vi "setParents.vi"(8 "error in (no error)":errorcluster, 10 "Parents":refnum<data-value>[](array[refnum]), 11 "MultiTreeNode in":refnum<class "MultiTreeNode.lvclass">) -> (0 "error out":errorcluster, 3 "MultiTreeNode out":refnum<class "MultiTreeNode.lvclass">)   [LabVIEW 2014, in "MultiTree.lvlib" / "MultiTreeNode.lvclass"]
uses:
  <userlib>/AdvancedDataStructures/ClassBased/MultiTreeNode/MultiTreeNode.lvclass
  <userlib>/AdvancedDataStructures/ClassBased/MultiTreeNode/MultiTreeNode.lvclass/MultiTreeNode.ctl
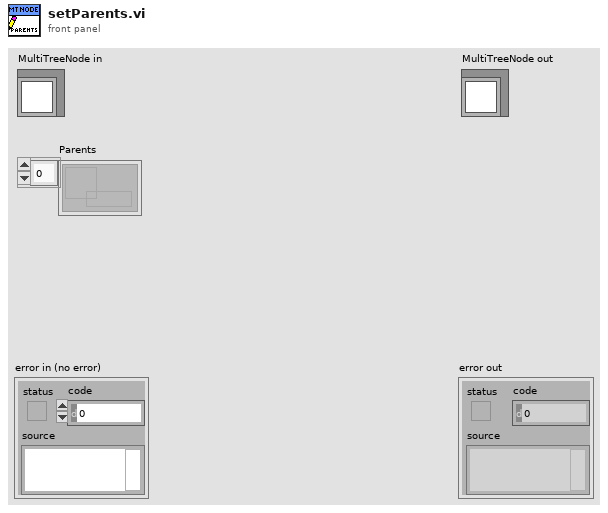
[diagram p1: front panel]
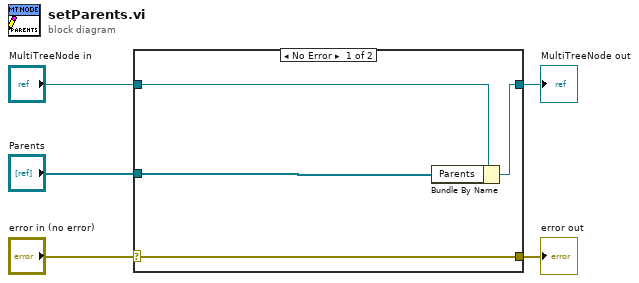
[diagram p0: block diagram]
diagram:
  n1 = case shown="No Error" "error in (no error)" {
    selector: "error in (no error)" -> [w9 w10]
    tunnel: [w9 w10] -> w4
    tunnel: [w7 w11] -> w2
    tunnel: "MultiTreeNode in" -> [w8 w11]
    tunnel: "Parents" -> [w6 _]
    frame No Error {
      n2 = Bundle By Name(cluster=w8, "Parents"=w6) -> (w7:refnum<class "MultiTreeNode.lvclass">)
    }
    frame Error {
    }
  }
  "error out" <- w4
  "MultiTreeNode out" <- w2
